vi "server.Parse Response (Numeric).vi"(8 "error in":errorcluster, 10 "Response String In":string) -> (0 "error out":errorcluster, 1 "LabVIEW Error?":bool=TRUE, 2 "value":dbl)   [LabVIEW 2016, in "JSONRPC Server.lvclass"]
uses:
  JSONRPC Server.lvclass
  <vilib>/NI/JSON Support for LabVIEW/JSON Data Classes/JSON Helper/To More Specific Type (Numeric).vi
  <vilib>/NI/JSON Support for LabVIEW/JSON Data Classes/JSON Numeric/Read value (Numeric).vi
  <vilib>/NI/JSON Support for LabVIEW/JSON Data Classes/JSON Helper/JSON Helper.lvclass
  <vilib>/NI/JSON Support for LabVIEW/JSON Data Classes/JSON Basic Type/JSON Literal.lvclass
  <vilib>/NI/JSON Support for LabVIEW/JSON Data Classes/JSON Numeric/JSON Numeric.lvclass
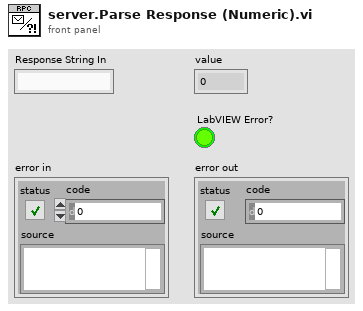
[diagram p1: front panel]
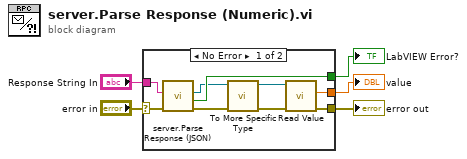
[diagram p0: block diagram]
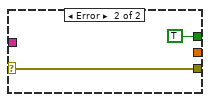
[diagram p2: hidden frame]
diagram:
  n1 = case shown="No Error" "error in" {
    selector: "error in" -> [w13 w16]
    tunnel: "Response String In" -> [w14 _]
    tunnel: [w12 TRUE ("LabVIEW Error?")] -> w3
    tunnel: [w8 _] -> w2
    tunnel: [w7 w16] -> w1
    frame No Error {
      n2 = call "server.Parse Response (JSON).vi"("error in"=w13, "Response String In"=w14) -> ("error out"=w10:errorcluster, "LabVIEW Error?"=w12:bool, "JSON out"=w11:refnum<class "JSON Null.lvclass">)  [unwired: 7 in]
      n3 = call-poly <vilib>:"To More Specific Type.vi"("error in (no error)"=w10, "JSON Datatype in"=w11) -> ("error out"=w6:errorcluster, "JSON Numeric out"=w9:refnum<class "JSON Numeric.lvclass">)  [unwired: 8 in]
      n4 = call-poly <vilib>:"Read Value.vi"("error in (no error)"=w6, "JSON Numeric in"=w9) -> ("error out"=w7:errorcluster, "value"=w8:dbl)  [unwired: 8 in]
    }
    frame Error {
    }
  }
  "error out" <- w1
  "LabVIEW Error?" <- w3
  "value" <- w2
